vi "getConnectionPoint.vi"(0 "reference":refnum<class "StateNode.lvclass">, 1 "direction":refnum<class "Direction.lvclass">, 5 "error in (no error)":errorcluster) -> (14 "reference out":refnum<class "StateNode.lvclass">, 15 "point2D":T1 {"y" format="%.2f"; "x" format="%.2f"}, 19 "error out":errorcluster)   [LabVIEW 2020, in "StateNode.lvclass"]
doc: "getConnectionPoint"
uses:
  <resource>/Framework/Providers/Open_GDS/UML/StateNode_class/StateNode.lvclass
  C:/Program Files (x86)/National Instruments/LabVIEW 2020/resource/Framework/Providers/Open_GDS/UML/RectangularNode_class/RectangularNode.lvclass
  <resource>/Framework/Providers/Open_GDS/UML/Direction_class/Direction.lvclass
  <resource>/Framework/Providers/Open_GDS/UML/General/Point/Point Point2D.ctl
  <resource>/Framework/Providers/Open_GDS/UML/RectangularNode_class/RectangularNode.lvclass
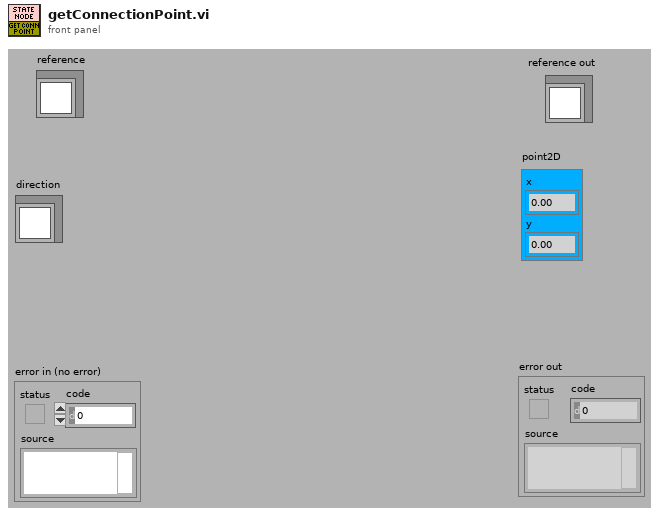
[diagram p1: front panel]
types:
  T1 = typedef "Point Point2D.ctl" = cluster{"x":dbl, "y":dbl}
  T2 = typedef "RectangularNode.lvclass/ObjectAttributes.ctl" = cluster{"bounds":T3}
  T3 = typedef "Rectangle Rectangle2D.ctl" = cluster{"x":dbl, "y":dbl, "width":dbl, "height":dbl}
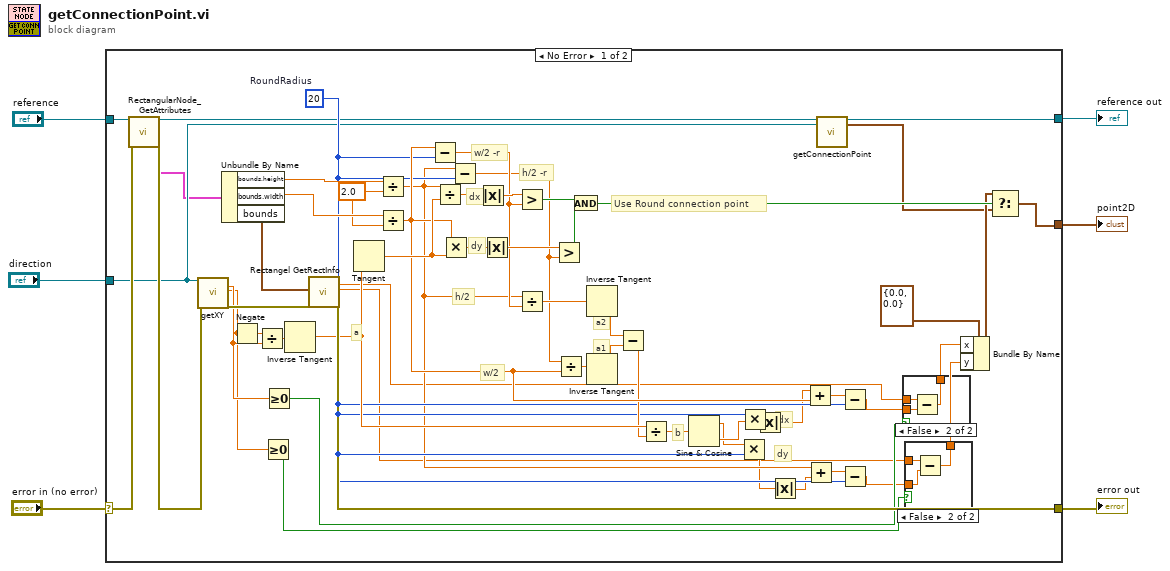
[diagram p0: block diagram]
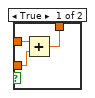
[diagram p2: hidden frame]
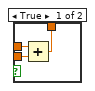
[diagram p3: hidden frame]
diagram:
  n1 = case shown="No Error" "error in (no error)" {
    selector: "error in (no error)" -> [w63 w76]
    tunnel: "reference" -> [w62 w77]
    tunnel: [w53 w76] -> w4
    tunnel: [w10 w77] -> w3
    tunnel: "direction" -> [w9 _]
    tunnel: [w42 _] -> w1
    frame No Error {
      w25 = i16 20  # RoundRadius
      w57 = 2.0 ("y")
      # "dy"
      # "dx"
      # "b"
      # "a"
      # "w/2"
      # "h/2 -r"
      # "a1"
      # "a2"
      # "h/2"
      # "w/2 -r"
      # "Use Round connection point"
      # "dy"
      # "dx"
      n2 = call <resource>:"RectangularNode_GetAttributes.vi"("reference in"=w62, "error in (no error)"=w63) -> ("reference out"=w11:refnum<class "StateNode.lvclass">, "Data"=w7:T2, "error out"=w61:errorcluster)  [unwired: 14 in, 1 out]
      n3 = call <resource>:"getXY.vi"("reference"=w9, "error in (no error)"=w61) -> ("x"=w52:dbl, "y"=w24:dbl, "error out"=w56:errorcluster)  [unwired: 15 out]
      n4 = Unbundle By Name(w7) -> ("bounds.height"=w59:dbl, "bounds.width"=w58:dbl, "bounds"=w55:T3)
      n5 = Negate(x=w24) -> (-x=w26:dbl)
      n6 = Divide(x=w26, y=w52) -> (x/y=w60:dbl)
      n7 = Greater Or Equal To 0?(x=w24) -> (x >= 0?=w12:bool)
      n8 = Greater Or Equal To 0?(x=w52) -> (x >= 0?=w21:bool)
      n9 = Inverse Tangent(1:w60) -> (0:w28:dbl)
      n10 = call <resource>:"Rectangel GetRectInfo.vi"("bounds"=w55, "error in (no error)"=w56) -> ("centerX"=w18:dbl, "centerY"=w14:dbl, "error out"=w53:errorcluster)  [unwired: 15 out]
      n11 = Tangent(1:w28) -> (0:w51:dbl)
      n12 = Divide(x=w59, y=w57) -> (x/y=w22:dbl)
      n13 = Divide(x=w58, y=w57) -> (x/y=w34:dbl)
      n14 = Subtract(x=w34, y=w25) -> (x-y=w41:dbl)
      n15 = Divide(x=w22, y=w51) -> (x/y=w50:dbl)
      n16 = Multiply(x=w34, y=w51) -> (x*y=w48:dbl)
      n17 = Subtract(x=w22, y=w25) -> (x-y=w39:dbl)
      n18 = Absolute Value(x=w50) -> (abs(x)=w49:dbl)
      n19 = Absolute Value(x=w48) -> (abs(x)=w47:dbl)
      n20 = Greater?(x=w49, y=w41) -> (0:w46:bool)
      n21 = Divide(x=w22, y=w41) -> (x/y=w40:dbl)
      n22 = Greater?(x=w47, y=w39) -> (0:w45:bool)
      n23 = Divide(x=w39, y=w34) -> (x/y=w38:dbl)
      n24 = And(x=w46, y=w45) -> (x .and. y?=w44:bool)
      n25 = Inverse Tangent(1:w40) -> (0:w37:dbl)
      n26 = Inverse Tangent(1:w38) -> (0:w36:dbl)
      n27 = Subtract(x=w37, y=w36) -> (x-y=w27:dbl)
      n28 = Divide(x=w28, y=w27) -> (x/y=w35:dbl)
      n29 = Sine & Cosine(0:w35) -> (1:w30:dbl, 2:w31:dbl)
      n30 = Multiply(x=w30, y=w25) -> (x*y=w20:dbl)
      n31 = Multiply(x=w25, y=w31) -> (x*y=w19:dbl)
      n32 = Absolute Value(x=w19) -> (abs(x)=w16:dbl)
      n33 = Absolute Value(x=w20) -> (abs(x)=w13:dbl)
      n34 = Add(x=w16, y=w34) -> (x+y=w33:dbl)
      n35 = Add(x=w22, y=w13) -> (x+y=w23:dbl)
      n36 = call-parent "getConnectionPoint.vi"("reference"=w11, "direction"=w9) -> ("reference out"=w10:refnum<class "StateNode.lvclass">, "point2D"=w8:T1)  [unwired: 15 in, 1 out]
      n37 = Subtract(x=w33, y=w25) -> (x-y=w17:dbl)
      n38 = Subtract(x=w23, y=w25) -> (x-y=w15:dbl)
      n39 = case shown="False" w21 {
        tunnel: w18 -> [w72 w75]
        tunnel: [w71 w74] -> w32
        tunnel: w17 -> [w70 w73]
        frame True {
          n40 = Add(x=w72, y=w70) -> (x+y=w71:dbl)
        }
        frame False {
          n41 = Subtract(x=w75, y=w73) -> (x-y=w74:dbl)
        }
      }
      n42 = case shown="False" w12 {
        tunnel: w14 -> [w66 w69]
        tunnel: w15 -> [w65 w68]
        tunnel: [w64 w67] -> w29
        frame True {
          n43 = Add(x=w66, y=w65) -> (x+y=w64:dbl)
        }
        frame False {
          n44 = Subtract(x=w69, y=w68) -> (x-y=w67:dbl)
        }
      }
      n45 = Bundle By Name(cluster=T1 {"x"=0.0, "y"=0.0} ("point2D"), "x"=w32, "y"=w29) -> (w43:T1)
      n46 = Select(t=w43, s=w44, f=w8) -> (s? t:f=w42:T1)
    }
    frame Error {
    }
  }
  "reference out" <- w3
  "error out" <- w4
  "point2D" <- w1
